vi "is image ready for update.vi"(9 "Last update":u32, 10 "min time between updates":u32, 11 "image ref in":T1) -> (3 "update image":bool)   [LabVIEW 2013]
uses:
  <vilib>/vision/Image Controls.llb/IMAQ Image.ctl
  <vilib>/vision/NI_Vision_Development_Module.lvlib
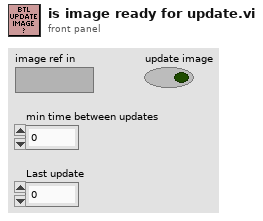
[diagram p1: front panel]
types:
  T1 = typedef "IMAQ Image.ctl" = refnum<image>
  T2 = cluster{"histogram":u32[], "Minimal Value":sgl, "Maximal Value":sgl, "Starting Value":sgl, "Interval Width":sgl, "Mean Value":sgl, "Standard  Variation":sgl, "Area (pixels)":i32}
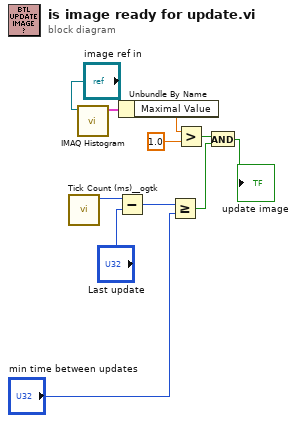
[diagram p0: block diagram]
diagram:
  n1 = call <userlib>:"Tick Count (ms)__ogtk.vi"() -> ("millisecond timer value"=w3:u32)  [unwired: 10 in, 1 out]
  n2 = call "IMAQ Histogram"("Image"="image ref in") -> ("Histogram Report"=w5:T2)  [unwired: 9 in, 1 out]
  n3 = Subtract(x=w3, y="Last update") -> (x-y=w2:u32)
  n4 = Unbundle By Name(w5) -> ("Maximal Value"=w6:sgl)
  n5 = Greater Or Equal?(x=w2, y="min time between updates") -> (x >= y?=w9:bool)
  n6 = Greater?(x=w6, y=sgl 1.0) -> (0:w8:bool)
  n7 = And(x=w8, y=w9) -> (x .and. y?=→"update image":bool)
